vi "usrp get rx rate.vi"(8 "error in (no error)":errorcluster, 9 "rate_out":dbl, 10 "chan":u64, 11 "h":u64) -> (0 "error out":errorcluster, 1 "rate_out out":dbl, 2 "function return":u32(ring), 3 "h 2":u64)   [LabVIEW 2023, in "uhd.lvlib"]
doc: "UHD_API uhd_error uhd_usrp_get_rx_rate(uhd_usrp_handle h, size_t chan, double* rate_out);"
uses:
  <userlib>/uhd/uhd.lvlib
  <userlib>/uhd/uhd.dll
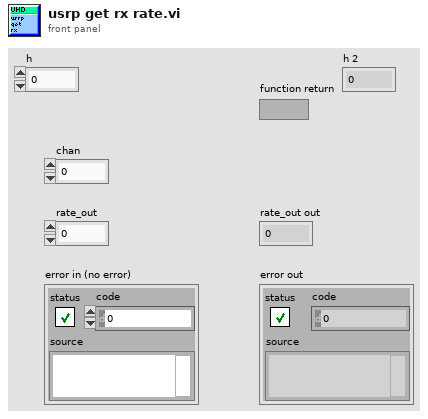
[diagram p1: front panel]
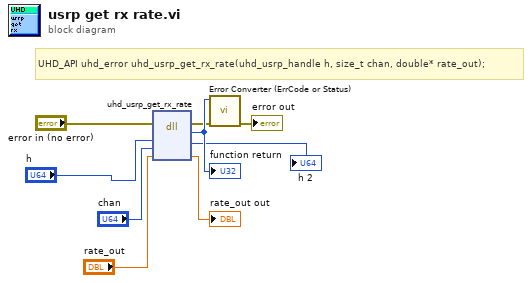
[diagram p0: block diagram]
diagram:
  # "UHD_API uhd_error uhd_usrp_get_rx_rate(uhd_usrp_handle h, size_t chan, double* rate_out);"
  n1 = dll-call lib="C:/Program Files/National Instruments/LabVIEW 2023/user.lib/uhd/uhd.dll" fn="uhd_usrp_get_rx_rate"(error in="error in (no error)", "h"="h", "chan"="chan", "rate_out"="rate_out") -> (error out=w4:errorcluster, "return type"=w9:u32, "h"=→"h 2":u64, "rate_out"=→"rate_out out":dbl)  [unwired: 3 in, 1 out]
  "function return" <- w9
  n2 = call <userlib>:"Error Converter (ErrCode or Status).vi"("error in (no error)"=w4, "error code"=w9) -> ("error out"=→"error out":errorcluster)  [unwired: 9 in]
